vi "resonant.display queue to fp display_rrMD.vi"() -> ()   [LabVIEW 2012]
doc: "SciScan 1.2 160622"
uses:
  <vilib>/Utility/VariantDataType/Type.ctl
  GFG/GFGnumericGet.vi
  GFG/GFGImageRefsGet.vi
  GFG/GFGDisplayRefsGet.vi
  GFG/GFGbooleanGet.vi
  GFG/GFG library.lvlib
  <vilib>/Utility/VariantDataType/VariantType.lvlib
panel:
  out "error out 3":errorcluster
  out "error out 2":errorcluster
  out "size(s)":i32[](array[numeric])
  out "# elements in display data queue":i32
  out "error out":errorcluster
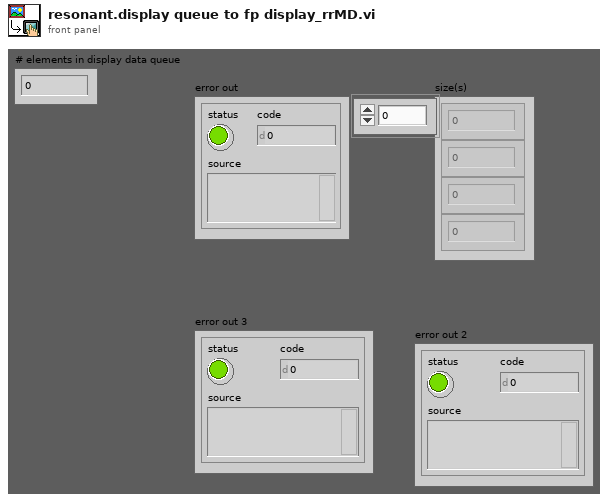
[diagram p1: front panel]
types:
  T1 = cluster{"Channel 1 small":refnum<vi>, "Channel 2 small":refnum<vi>, "Channel 3 small":refnum<vi>, "Channel 4 small":refnum<vi>, "Channel 1 large":refnum<vi>, "Channel 2 large":refnum<vi>, "Channel 3 large":refnum<vi>, "Channel 4 large":refnum<vi>, "RGB overlay":refnum<vi>, "ROI Image display":refnum<vi>, "arb line scan display":refnum<vi>, "Channel 5 large":refnum<vi>}
  T2 = typedef "IMAQ Image.ctl" = refnum<image>
  T3 = cluster{"Channel 1 small":T2, "Channel 2 small":T2, "Channel 3 small":T2, "Channel 4 small":T2, "Channel 1 large":T2, "Channel 2 large":T2, "Channel 3 large":T2, "Channel 4 large":T2, "RGB overlay":T2, "ROI Image display":T2, "arb line scan display":T2, "Channel 5 large":T2}
  T4 = cluster{"NewVal":bool, "Event Registration Refnum":refnum<event-registration>}
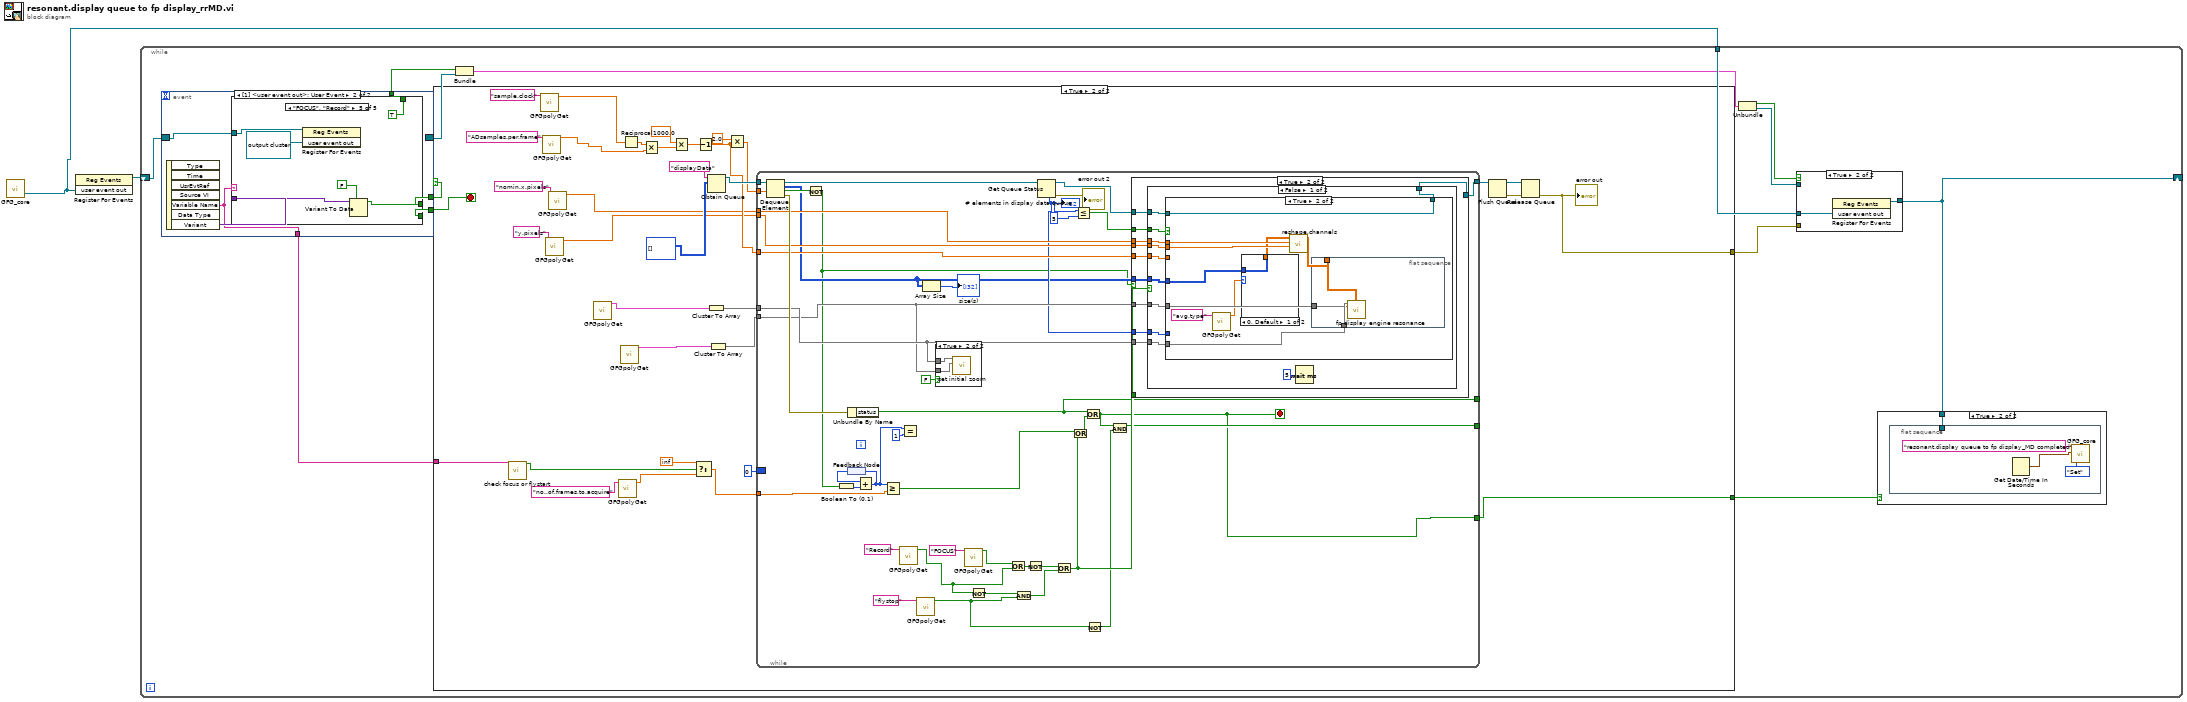
[diagram p0: block diagram]
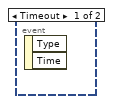
[diagram p4: hidden frame]
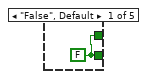
[diagram p5: hidden frame]
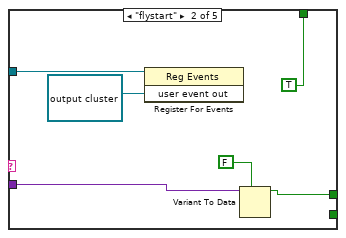
[diagram p6: hidden frame]
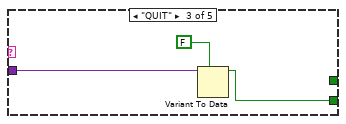
[diagram p7: hidden frame]
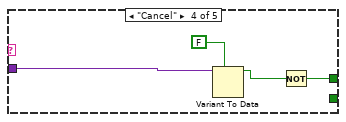
[diagram p8: hidden frame]
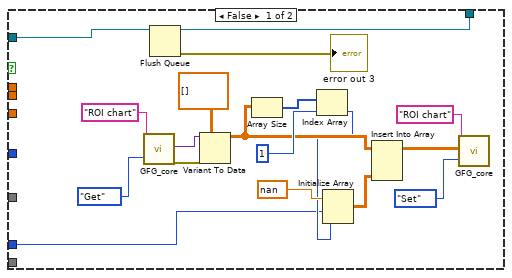
[diagram p11: hidden frame]
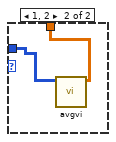
[diagram p12: hidden frame]
diagram:
  n1 = call "GFG_core.vi"() -> ("user event out"=w2:refnum<user-event>)  [unwired: 13 in, 6 out]
  n2 = register-events(w2) -> (reference out=w1:refnum<event-registration>)  [unwired: 2 in, 1 out]
  n3 = while {
    shift-right: [w3] -> _
    shift-left: w1 -> [w11]
    tunnel: w2 -> [w13]
    stop <- w14 stop-if-true
    n4 = event shown="[1] <user event out>: User Event" {
      selector: w11 -> [_ w24]
      dyn-events: [_ _] -> w9
      timeout: _ -> [_ _]
      tunnel: [_ w28] -> w15
      tunnel: [_ w27] -> w14
      tunnel: [_ w25] -> w5
      tunnel: [_ w23] -> w10
      event Timeout {
        n5 = event-data() -> ()  [unwired: 1 in, 2 out]
      }
      event User Event {
        n6 = event-data() -> ("Variable Name"=w25:string, "Variant"=w26:variant)  [unwired: 1 in, 5 out]
        n7 = case shown="\"FOCUS\", \"Record\"" w25 {
          tunnel: [w29 w33 _ w39 w46] -> w28
          tunnel: [w29 _ w36 _ _] -> w27
          tunnel: w26 -> [_ w34 w38 w41 w47]
          tunnel: w24 -> [_ w31 _ _ w44]
          tunnel: [_ TRUE ("NewVal") _ _ TRUE ("NewVal")] -> w23
          frame "False", Default {
            w29 = FALSE ("NewVal")
          }
          frame "flystart" {
            n8 = register-events(reference=w31, refnum<user-event> refnum ("user event out")) -> ()  [unwired: 1 in, 2 out]
            n9 = Variant To Data(type=FALSE ("NewVal"), Variant=w34) -> (data=w33:bool)  [unwired: 1 in, 1 out]
          }
          frame "QUIT" {
            n10 = Variant To Data(type=FALSE ("NewVal"), Variant=w38) -> (data=w36:bool)  [unwired: 1 in, 1 out]
          }
          frame "Cancel" {
            n11 = Variant To Data(type=FALSE ("NewVal"), Variant=w41) -> (data=w40:bool)  [unwired: 1 in, 1 out]
            n12 = Not(x=w40) -> (.not. x?=w39:bool)
          }
          frame "FOCUS", "Record" {
            n13 = register-events(reference=w44, refnum<user-event> refnum ("user event out")) -> ()  [unwired: 1 in, 2 out]
            n14 = Variant To Data(type=FALSE ("NewVal"), Variant=w47) -> (data=w46:bool)  [unwired: 1 in, 1 out]
          }
        }
      }
    }
    n15 = case shown="True" w15 {
      tunnel: [_ w54] -> w12
      tunnel: w5 -> [_ w56]
      tunnel: [_ w52] -> w4
      frame False {
      }
      frame True {
        n16 = call "check focus or flystart.vi"("GFG variable name"=w56) -> ("Focus or flystart?"=w55:bool)  [unwired: 10 in]
        n17 = call-poly "GFGpolyGet.vi"("Variable Name in"="sample.clock" ("Tag in")) -> ("Numeric"=w74:dbl)  [unwired: 8 in, 2 out]
        n18 = call-poly "GFGpolyGet.vi"("Variable Name in"="ADsamples.per.frame" ("Tag in")) -> ("Numeric"=w62:dbl)  [unwired: 8 in, 2 out]
        n19 = call-poly "GFGpolyGet.vi"("Variable Name in"="y.pixels") -> ("Numeric"=w50:dbl)  [unwired: 8 in, 2 out]
        n20 = call-poly "GFGpolyGet.vi"("Variable Name in"="nomin.x.pixels") -> ("Numeric"=w51:dbl)  [unwired: 8 in, 2 out]
        n21 = call-poly "GFGpolyGet.vi"() -> ("DisplayRefsOut(generic class)"=w71:T1)  [unwired: 10 in, 1 out]
        n22 = call-poly "GFGpolyGet.vi"("Variable Name in"="no..of.frames.to.acquire" ("Tag in")) -> ("Numeric"=w58:dbl)  [unwired: 8 in, 2 out]
        n23 = call-poly "GFGpolyGet.vi"() -> ("Image Refs Out"=w70:T3)  [unwired: 10 in, 1 out]
        n24 = Reciprocal(x=w74) -> (1/x=w79:dbl)
        n25 = Multiply(x=w79, y=w62) -> (x*y=w78:dbl)
        n26 = Multiply(x=1000.0, y=w78) -> (x*y=w76:dbl)
        n27 = Select(t=inf, s=w55, f=w58) -> (s? t:f=w57:dbl)
        n28 = Decrement(x=w76) -> (x-1=w61:dbl)
        n29 = Obtain Queue(name (unnamed)="displayData", element data type=i16[][] [] ("initialized array")) -> (queue out=w72:refnum<queue>)  [unwired: 3 in, 2 out]
        n30 = Cluster To Array(cluster=w71) -> (array=w68:refnum<vi>[])
        n31 = Cluster To Array(cluster=w70) -> (array=w69:T2[])
        n32 = Multiply(x=2.0, y=w61) -> (x*y=w67:dbl)
        n33 = while {
          tunnel: [w108] -> w65
          tunnel: w57 -> [w88]
          tunnel: w67 -> [w122]
          tunnel: w72 -> [w123]
          tunnel: w68 -> [w118]
          tunnel: w69 -> [w113]
          tunnel: w51 -> [w111]
          tunnel: w50 -> [w110]
          tunnel: w61 -> [w117]
          tunnel: [w102] -> w52
          tunnel: [w105] -> _
          tunnel: [w101] -> _
          border: i16 0 -> [_]
          stop <- w102 stop-if-true
          n34 = Dequeue Element(queue=w123, timeout in ms (-1)=w122) -> (queue out=w121:refnum<queue>, element=w100:i16[][], timed out?=w114:bool, error out=w124:errorcluster)  [unwired: 1 in]
          n35 = Not(x=w114) -> (.not. x?=w84:bool)
          n36 = Boolean To (0,1)(Boolean=w84) -> (0, 1=w90:i16)
          n37 = Unbundle By Name(w124) -> ("status"=w101:bool)
          n38 = feedback #1() -> (w89:i16)
          n39 = Add(x=w89, y=w90) -> (x+y=w86:i16)
          n40 = feedback-in #1(w86) -> ()
          n41 = Greater Or Equal?(x=w86, y=w88) -> (x >= y?=w87:bool)
          n42 = call-poly "GFGpolyGet.vi"("Variable Name in"="Record") -> ("Boolean Value OUT"=w92:bool)  [unwired: 9 in, 1 out]
          n43 = Equal?(x=w86, y=1) -> ()  [unwired: 1 out]
          n44 = call-poly "GFGpolyGet.vi"("Variable Name in"="flystop") -> ("Boolean Value OUT"=w104:bool)  [unwired: 9 in, 1 out]
          n45 = Array Size(array=w100) -> (size(s)=→"size(s)":i32[])
          n46 = case shown="True" FALSE {
            tunnel: w118 -> [_ w184]
            tunnel: w113 -> [_ w183]
            frame False {
            }
            frame True {
              n47 = call "set initial zoom.vi"("Image Refs In"=w183, "DisplayRefsIn(generic class)"=w184) -> ()  [unwired: 10 in]
            }
          }
          n48 = call-poly "GFGpolyGet.vi"("Variable Name in"="FOCUS") -> ("Boolean Value OUT"=w98:bool)  [unwired: 9 in, 1 out]
          n49 = Not(x=w92) -> (.not. x?=w93:bool)
          n50 = Or(x=w98, y=w92) -> (x .or. y?=w99:bool)
          n51 = And(x=w93, y=w104) -> (x .and. y?=w91:bool)
          n52 = Not(x=w99) -> (.not. x?=w95:bool)
          n53 = Get Queue Status(queue=w121) -> (queue out=w109:refnum<queue>, error out=→"error out 2":errorcluster, # elements in queue=w107:i32)  [unwired: 2 in, 5 out]
          "# elements in display data queue" <- w107
          n54 = Or(x=w95, y=w91) -> (x .or. y?=w120:bool)
          n55 = Or(x=w87, y=w120) -> (x .or. y?=w106:bool)
          n56 = Less Or Equal?(x=w107, y=5) -> (x <= y?=w85:bool)
          n57 = Or(x=w101, y=w106) -> (x .or. y?=w102:bool)
          n58 = Not(x=w104) -> (.not. x?=w103:bool)
          n59 = And(x=w102, y=w103) -> (x .and. y?=w105:bool)
          n60 = case shown="True" w84 {
            tunnel: w120 -> [_ w136]
            tunnel: w118 -> [_ w135]
            tunnel: w117 -> [_ w134]
            tunnel: w113 -> [_ w133]
            tunnel: w111 -> [_ w132]
            tunnel: w110 -> [_ w131]
            tunnel: w109 -> [w125 w130]
            tunnel: [w125 w129] -> w108
            tunnel: w107 -> [_ w128]
            tunnel: w100 -> [_ w127]
            tunnel: w85 -> [_ w126]
            frame False {
            }
            frame True {
              n61 = case shown="False" w136 {
                tunnel: w132 -> [w147 _]
                tunnel: w131 -> [w146 _]
                tunnel: w127 -> [w145 _]
                tunnel: w135 -> [w144 _]
                tunnel: w133 -> [w143 _]
                tunnel: w134 -> [w142 _]
                tunnel: w126 -> [w141 _]
                tunnel: w130 -> [w140 w182]
                tunnel: [w139 w182] -> w129
                tunnel: w128 -> [w138 _]
                frame False {
                  n62 = case shown="True" w141 {
                    tunnel: w147 -> [_ w175]
                    tunnel: w146 -> [_ w174]
                    tunnel: w145 -> [_ w173]
                    tunnel: w144 -> [_ w171]
                    tunnel: w143 -> [_ w170]
                    tunnel: w142 -> [_ _]
                    tunnel: w140 -> [w152 w169]
                    tunnel: [w150 w169] -> w139
                    tunnel: w138 -> [w148 _]
                    frame False {
                      n63 = call "GFG_core.vi"("Variable Name in"="ROI chart", "Action"=enum16{"Init", "Set", "Get"}."Get") -> ("Variant Out"=w162:variant, "error out"=w163:errorcluster)  [unwired: 11 in, 5 out]
                      n64 = Flush Queue(queue=w152) -> (queue out=w150:refnum<queue>, error out=→"error out 3":errorcluster)  [unwired: 1 in, 1 out]
                      n65 = Variant To Data(error in=w163, type=sgl[][] [] ("y backward image"), Variant=w162) -> (data=w158:sgl[][])  [unwired: 1 out]
                      n66 = Array Size(array=w158) -> (size(s)=w156:i32[])
                      n67 = Index Array(array=w156, index=1) -> (element=w149:i32)
                      n68 = Initialize Array(nan, w148, w149) -> (w157:dbl[][])
                      n69 = Insert Into Array(array=w158, new element=w157) -> (w153:sgl[][])  [unwired: 2 in]
                      n70 = call "GFG_core.vi"("Variable Name in"="ROI chart", "Variant in"=w153, "Action"=enum16{"Init", "Set", "Get"}."Set") -> ()  [unwired: 10 in, 7 out]
                    }
                    frame True {
                      n71 = call-poly "GFGpolyGet.vi"("Variable Name in"="avg.type") -> ("Numeric"=w166:dbl)  [unwired: 8 in, 2 out]
                      n72 = case shown="0, Default" w166 {
                        tunnel: w173 -> [w179 w181]
                        tunnel: [w179 w180] -> w172
                        frame 0, Default {
                        }
                        frame 1, 2 {
                          n73 = call "avgvi.vi"("image in"=w181) -> ("image out"=w180:sgl[][])  [unwired: 10 in]
                        }
                      }
                      n74 = call "reshape.channels.vi"("y.pixels"=w174, "x.pixels"=w175, "element"=w172) -> ("Array"=w168:dbl[][][])  [unwired: 8 in]
                      n75 = flat-sequence {
                        tunnel: w168 -> [w178]
                        tunnel: w171 -> [w177]
                        tunnel: w170 -> [w176]
                        frame #0 {
                          n76 = call "fp display engine resonance.vi"("channel data in"=w178, "Image Refs In"=w176, "DisplayRefsIn(generic class)"=w177) -> ()  [unwired: 9 in]
                        }
                      }
                    }
                  }
                  n77 = Wait (ms)(milliseconds to wait=u32 5) -> ()  [unwired: 1 out]
                }
                frame True {
                }
              }
            }
          }
        }
        n78 = Flush Queue(queue=w65) -> (queue out=w82:refnum<queue>, error out=w81:errorcluster)  [unwired: 1 in, 1 out]
        n79 = Release Queue(queue=w82, error in (no error)=w81) -> (error out=w54:errorcluster)  [unwired: 1 in, 2 out]
        "error out" <- w54
      }
    }
    n80 = Bundle("NewVal"=w10, "Event Registration Refnum"=w9) -> (w8:T4)  [unwired: 1 in]
    n81 = Unbundle(w8) -> ("NewVal"=w7:bool, "Event Registration Refnum"=w6:refnum<event-registration>)
    n82 = case shown="True" w7 {
      tunnel: [w20 w22] -> w3
      tunnel: w13 -> [_ w21]
      tunnel: w12 -> [_ _]
      tunnel: w6 -> [w20 _]
      frame False {
      }
      frame True {
        n83 = register-events(w21) -> (reference out=w22:refnum<event-registration>)  [unwired: 2 in, 1 out]
      }
    }
    n84 = case shown="True" w4 {
      tunnel: w3 -> [_ w16]
      frame False {
      }
      frame True {
        n85 = flat-sequence {
          tunnel: w16 -> [_]
          frame #0 {
            n86 = Get Date/Time In Seconds() -> (seconds since 1Jan1904=w17:timestamp)
            n87 = call "GFG_core.vi"("Variable Name in"="resonant.display queue to fp display_MD completed", "Variant in"=w17, "Action"=enum16{"Init", "Set", "Get"}."Set") -> ()  [unwired: 10 in, 7 out]
          }
        }
      }
    }
  }
